vi "Read QR Code(1).vi"(11 "error in (no error)":errorcluster) -> (2 "error out":errorcluster, 3 "Image Value":i32)   [LabVIEW 2018]
doc: "The myRIO Project template acquires acceleration data from the onboard accelerometer and displays the changes of acceleration values in a waveform chart."
uses:
  <vilib>/myRIO/Instrument Drivers/Onboard IO/UART/typedef/VISA Configuration.ctl
  <vilib>/Instr/_visa.llb/VISA Configure Serial Port (Instr).vi
  <vilib>/myRIO/Express VI/Onboard IO/UART/UART Express VI.xnode
  <vilib>/myRIO/Instrument Drivers/Onboard IO/UART/UART.lvlib
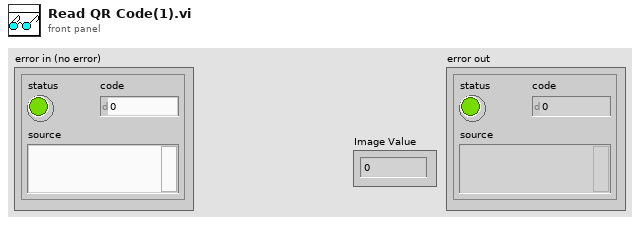
[diagram p1: front panel]
types:
  T1 = typedef "UART.lvlib/VISA Configuration.ctl" = cluster{"baud rate (9600)":u32, "data bits (8)":u16, "parity (0:none)":enum16{"None", "Odd", "Even", "Mark", "Space"}, "stop bits (10: 1 bit)":u16, "flow control (0:none)":u16, "termination char\n(0xA = '\\n' = LF) ":u8, "Enable Termination\nChar (T)":bool, "timeout (10sec)":u32}
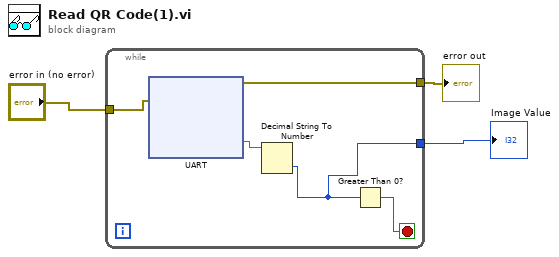
[diagram p0: block diagram]
diagram:
  n1 = while {
    tunnel: [w6] -> w3
    tunnel: "error in (no error)" -> [w5]
    tunnel: [w4] -> w1
    stop <- w7 stop-if-true
    n2 = xnode "UART"("error in (no error)"=w5) -> ("Characters Read"=w8:string, "error out"=w4:errorcluster)
    n3 = Decimal String To Number(string=w8) -> (number=w6:i32)  [unwired: 2 in, 1 out]
    n4 = Greater Than 0?(x=w6) -> (x > 0?=w7:bool)
  }
  "Image Value" <- w3
  "error out" <- w1
